vi "New Data Logging Specification.vi"   [LabVIEW 2020, in "NI_VS Data Logging API.lvlib"]
doc: "Creates a new data logging specification, which defines the channels to log and the type and base path for log files. You can log data to TDMS or text (.txt) files. You must manually select the polymorphic instance to use."
uses:
  <vilib>/NI VeriStand/Execution/DataLogging/NI_VS Data Logging API.lvlib
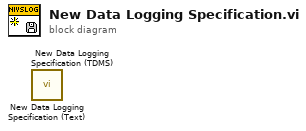
[diagram p0: block diagram]
diagram:
  n1 = call <vilib>:"New Data Logging Specification (Text).vi"() -> ()  [unwired: 10 in, 2 out]
  n2 = call <vilib>:"New Data Logging Specification (TDMS).vi"() -> ()  [unwired: 10 in, 2 out]
